vi "Striker.vi"(4 "balls":T4[](array[typedef]), 6 "geometry":T5, 8 "atacando ao contrário?":bool=TRUE, 9 "IA Input":T1, 10 "Robot":T2, 11 "command\nenum":T7) -> (2 "output cluster":T2)   [LabVIEW 2016]
uses:
  Core/AI Robot.ctl
  Functions Enum.ctl
  Command Enum.ctl
  Core/Field Size.ctl
  Core/AI Ball.ctl
  Core/AI Input.ctl
  Core/AI Judge.ctl
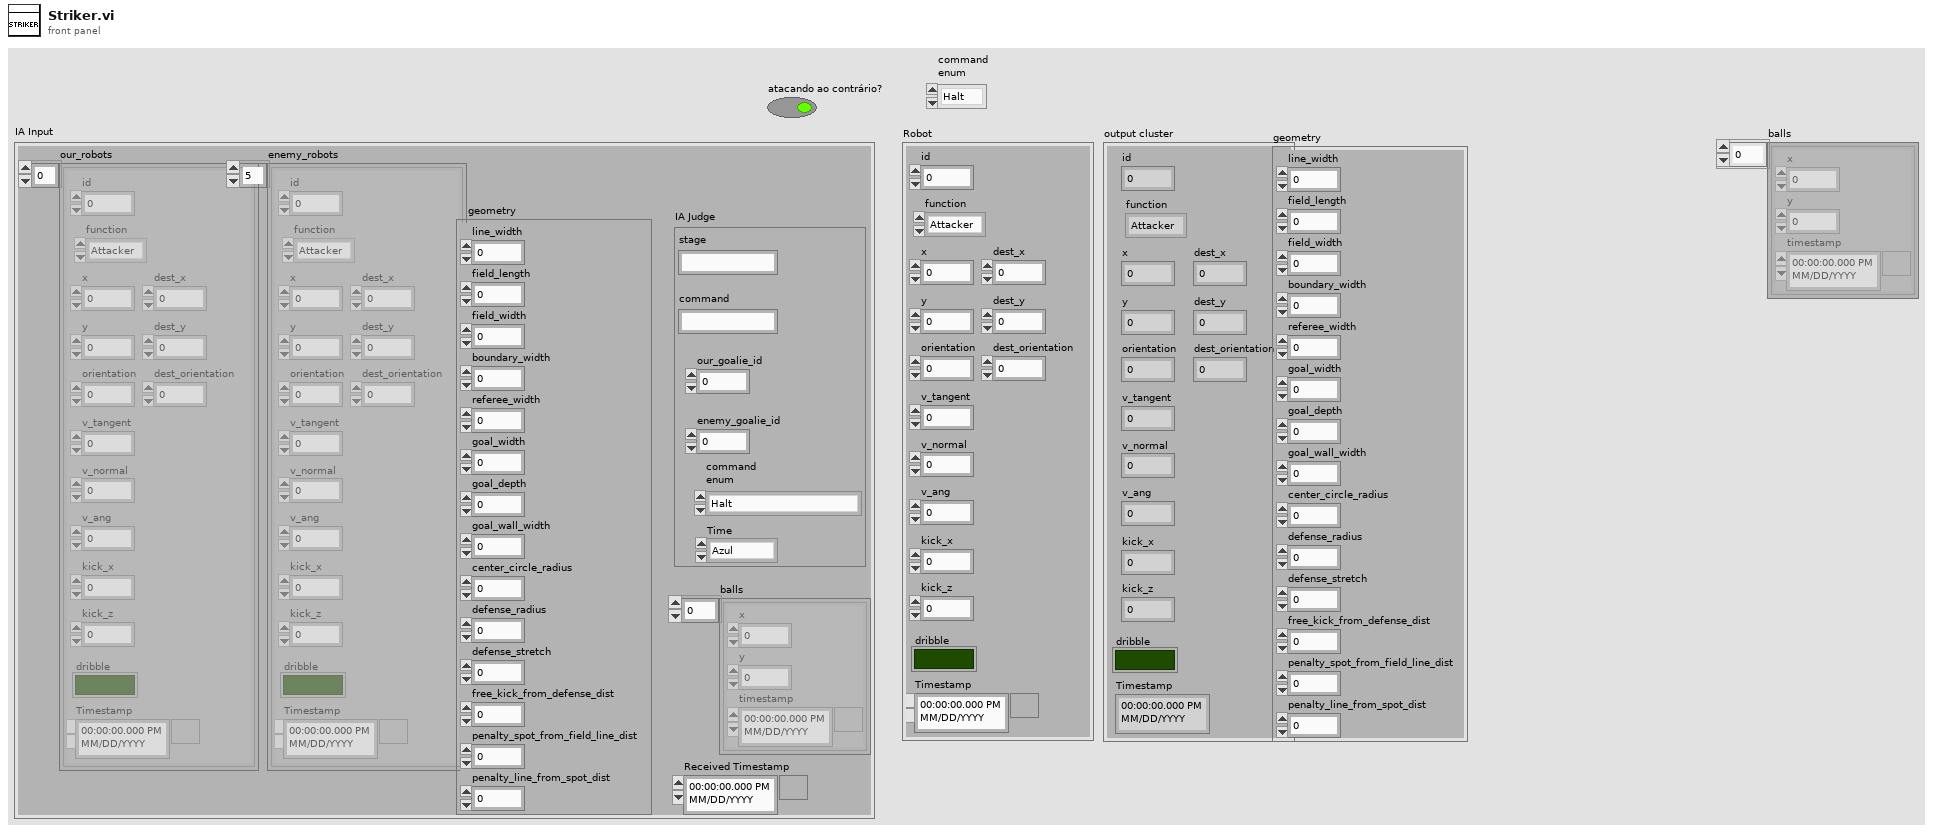
[diagram p1: front panel]
types:
  T1 = typedef "AI Input.ctl" = cluster{"our_robots":T2[], "enemy_robots":T2[], "balls":T4[], "geometry":T5, "IA Judge":T6, "Received Timestamp":timestamp}
  T2 = typedef "AI Robot.ctl" = cluster{"id":u32, "function":T3, "x":dbl, "y":dbl, "orientation":dbl, "v_tangent":dbl, "v_normal":dbl, "v_ang":dbl, "kick_x":dbl, "kick_z":dbl, "dribble":bool, "Timestamp":timestamp, "dest_x":dbl, "dest_y":dbl, "dest_orientation":dbl}
  T3 = typedef "Functions Enum.ctl" = enum16{"Attacker", "Goalie", "Defender", "Striker", "Goto 0", "Dummy", "ZigZag"}
  T4 = typedef "AI Ball.ctl" = cluster{"x":dbl, "y":dbl, "timestamp":timestamp}
  T5 = typedef "Field Size.ctl" = cluster{"line_width":u32, "field_length":u32, "field_width":u32, "boundary_width":u32, "referee_width":u32, "goal_width":u32, "goal_depth":u32, "goal_wall_width":u32, "center_circle_radius":u32, "defense_radius":u32, "defense_stretch":u32, "free_kick_from_defense_dist":u32, "penalty_spot_from_field_line_dist":u32, "penalty_line_from_spot_dist":u32}
  T6 = typedef "AI Judge.ctl" = cluster{"stage":string, "command":string, "our_goalie_id":dbl, "enemy_goalie_id":dbl, "command\nenum":T7, "Time":enum16{"Azul", "Amarelo"}}
  T7 = typedef "Command Enum.ctl" = enum16{"Halt", "Stop", "Force Start", "PKA Normal Start", "Prepare Kickoff Ally", "PKE Normal Start", "Prepare Kickoff Enemy", "Prepare Penalty Ally", "PPA Normal Start", "Prepare Penalty Enemy", "PPE Normal Start", "Direct Free Enemy", "Direct Free Ally", "Indirect Free Enemy", "Indirect Free Ally", "Timeout Enemy", "Timeout Ally", "Goal Enemy", "Goal Ally", "Ball Placement Enemy", "Ball Placement Ally", "None"}
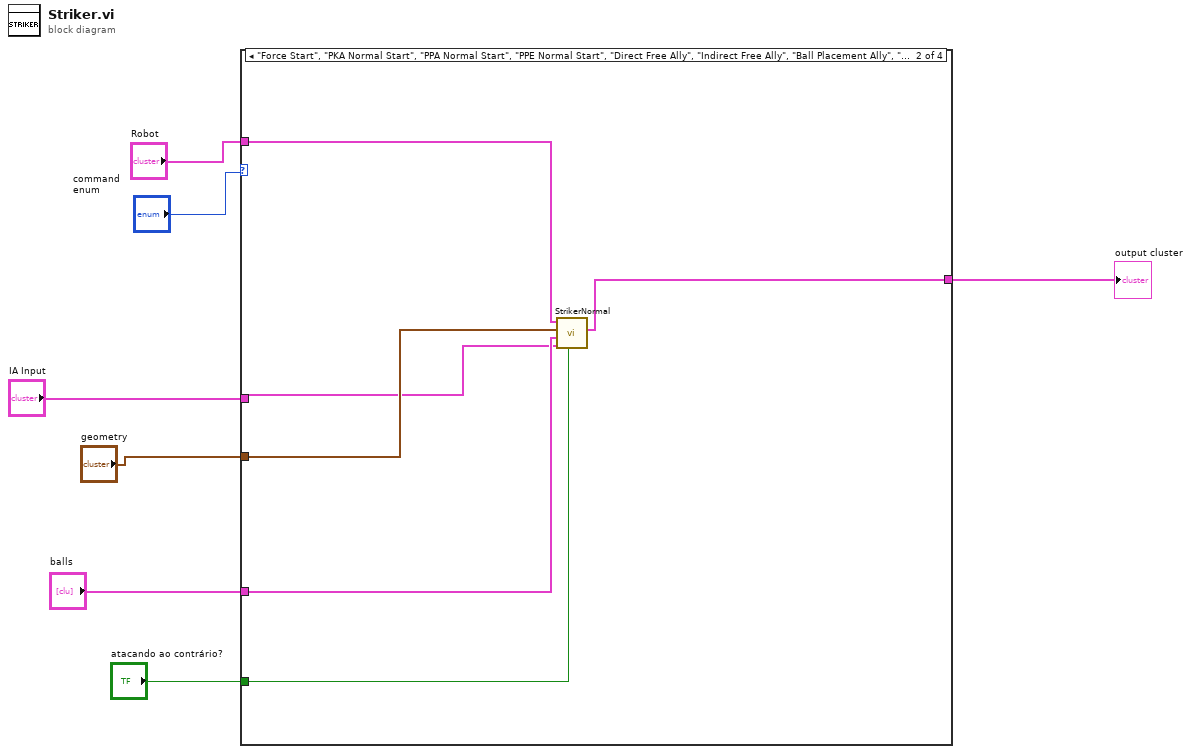
[diagram p0: block diagram]
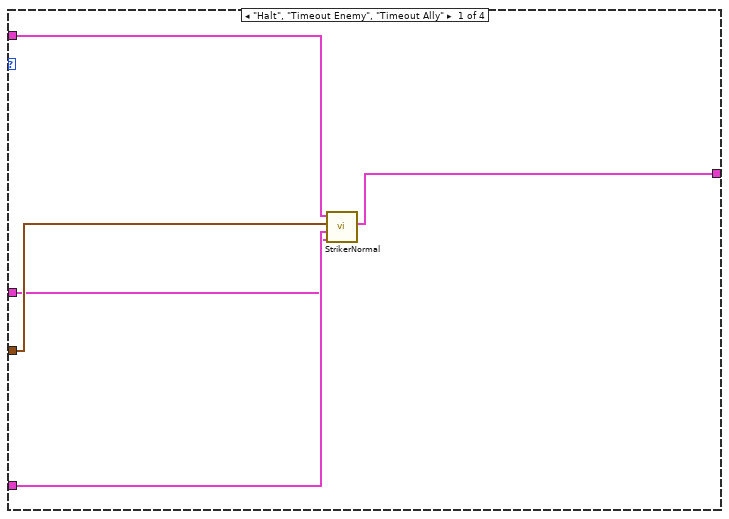
[diagram p2: hidden frame]
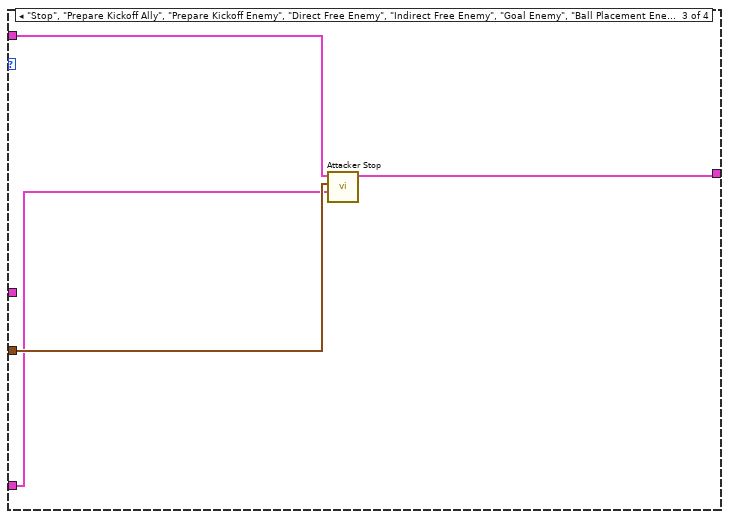
[diagram p3: hidden frame]
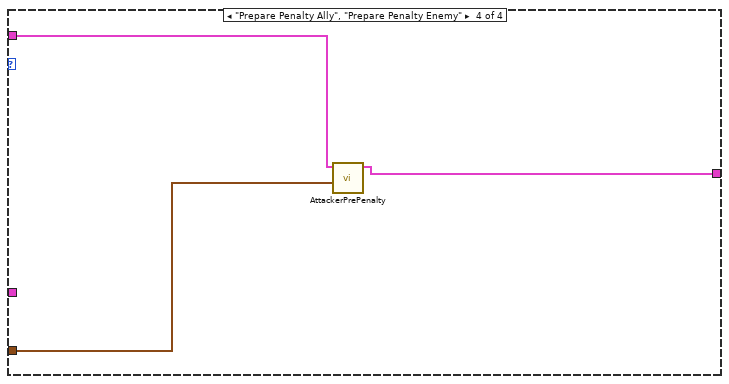
[diagram p4: hidden frame]
diagram:
  n1 = case shown="\"Force Start\", \"PKA Normal Start\", \"PPA Normal Start\", \"PPE Normal Start\", \"Direct Free Ally\", \"Indirect Free Ally\", \"Ball Placement Ally\", \"None\", Default" "command\nenum" {
    tunnel: "Robot" -> [w11 w15 w22 w25]
    tunnel: [w12 w18 w19 w23] -> w5
    tunnel: "geometry" -> [w10 w16 w21 w24]
    tunnel: "balls" -> [w9 w17 w20 _]
    tunnel: "IA Input" -> [w8 w14 _ _]
    tunnel: "atacando ao contrário?" -> [_ w13 _ _]
    frame "Halt", "Timeout Enemy", "Timeout Ally" {
      n2 = call "StrikerNormal.vi"("IA Input"=w8, "balls"=w9, "Field Size in"=w10, "Robot in"=w11) -> ("Robot out"=w12:T2)  [unwired: 7 in]
    }
    frame "Force Start", "PKA Normal Start", "PPA Normal Start", "PPE Normal Start", "Direct Free Ally", "Indirect Free Ally", "Ball Placement Ally", "None", Default {
      n3 = call "StrikerNormal.vi"("atacando ao contrário?"=w13, "IA Input"=w14, "balls"=w17, "Field Size in"=w16, "Robot in"=w15) -> ("Robot out"=w18:T2)  [unwired: 6 in]
    }
    frame "Stop", "Prepare Kickoff Ally", "Prepare Kickoff Enemy", "Direct Free Enemy", "Indirect Free Enemy", "Goal Enemy", "Ball Placement Enemy" {
      n4 = call "Attacker Stop.vi"("balls"=w20, "Field Size in"=w21, "Robot in"=w22) -> ("Robot out"=w19:T2)  [unwired: 8 in]
    }
    frame "Prepare Penalty Ally", "Prepare Penalty Enemy" {
      n5 = call "AttackerPrePenalty.vi"("Field Size in"=w24, "Robot in"=w25) -> ("Robot out"=w23:T2)  [unwired: 9 in]
    }
  }
  "output cluster" <- w5
